vi "停止整机测试(子VI).vi"   [LabVIEW 2016]
types:
  T1 = cluster{"命令":string, cluster{"starting address":u16, "holding register value":u16}}
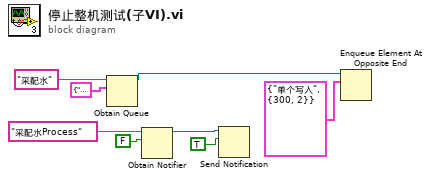
[diagram p0: block diagram]
diagram:
  n1 = Obtain Queue(name (unnamed)="采配水" ("名称（未命名）"), element data type=cluster{"命令":string, "数据":variant} {"命令"="", "数据"=variant}) -> (queue out=w6:refnum<queue>)  [unwired: 3 in, 2 out]
  n2 = Obtain Notifier(name (unnamed)="采配水Process" ("名称（未命名）"), notification data type=FALSE) -> (notifier out=w8:refnum<notifier>)  [unwired: 2 in, 2 out]
  n3 = Send Notification(notification=TRUE ("通知"), notifier=w8) -> ()  [unwired: 1 in, 2 out]
  n4 = Enqueue Element At Opposite End(queue=w6, element=T1 {"命令"="单个写入", {"starting address"=300, "holding register value"=2}} ("元素")) -> ()  [unwired: 2 in, 3 out]
